vi "current time (HHMMSS.SSS-to-SSSSS.SSS).vi"() -> (3 "Numeric":dbl)   [LabVIEW 2024]
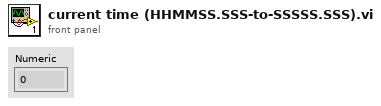
[diagram p1: front panel]
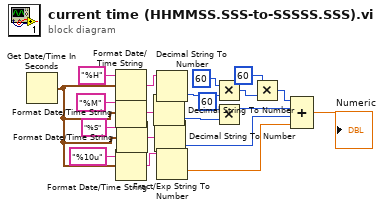
[diagram p0: block diagram]
diagram:
  n1 = Get Date/Time In Seconds() -> (seconds since 1Jan1904=w1:timestamp)
  n2 = Format Date/Time String(time format string (%c)="%H", seconds (now)=w1) -> (date/time string=w3:string)  [unwired: 1 in]
  n3 = Format Date/Time String(time format string (%c)="%M", seconds (now)=w1) -> (date/time string=w4:string)  [unwired: 1 in]
  n4 = Format Date/Time String(time format string (%c)="%10u", seconds (now)=w1) -> (date/time string=w2:string)  [unwired: 1 in]
  n5 = Format Date/Time String(time format string (%c)="%S", seconds (now)=w1) -> (date/time string=w5:string)  [unwired: 1 in]
  n6 = Decimal String To Number(string=w4) -> (number=w6:i32)  [unwired: 2 in, 1 out]
  n7 = Decimal String To Number(string=w5) -> (number=w9:i32)  [unwired: 2 in, 1 out]
  n8 = Decimal String To Number(string=w3) -> (number=w7:i32)  [unwired: 2 in, 1 out]
  n9 = Fract/Exp String To Number(string=w2) -> (number=w12:dbl)  [unwired: 3 in, 1 out]
  n10 = Multiply(x=60, y=w7) -> (x*y=w8:i32)
  n11 = Multiply(x=60, y=w6) -> (x*y=w10:i32)
  n12 = Multiply(x=60, y=w8) -> (x*y=w11:i32)
  n13 = Compound Arithmetic op=ADD(w11, w10, w9, w12) -> (→"Numeric":dbl)
